vi "CDEx Draw Helicopter 3D Model.vi"(7 "Reset?":bool, 9 "Pitch":dbl, 10 "Travel":dbl, 11 "Elevation":dbl) -> (3 "Scene.New Object":refnum<vi>)   [LabVIEW 2015]
doc: "This VI draws the Flexible Joint using the \"LabVIEW 3D Picture Control Evaluation Software\".\nThe evaluation software can be downloaded from the following URL: http://digital.ni.com/express.nsf/express?openagent&code=exn4gy"
uses:
  <vilib>/picture/3D Picture Control/NI_3D Picture Control.lvlib
panel:
  out "3D Picture Control":refnum<vi>(3d-picture)
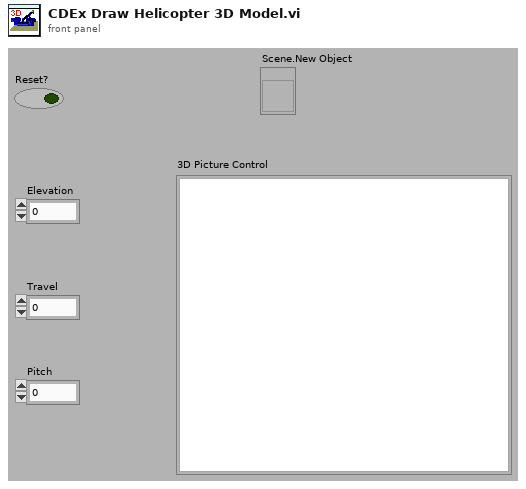
[diagram p1: front panel]
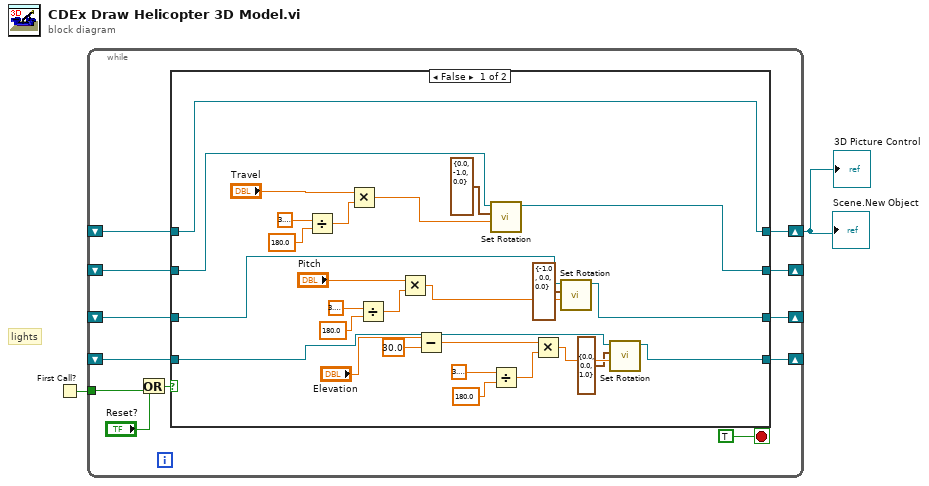
[diagram p0: block diagram]
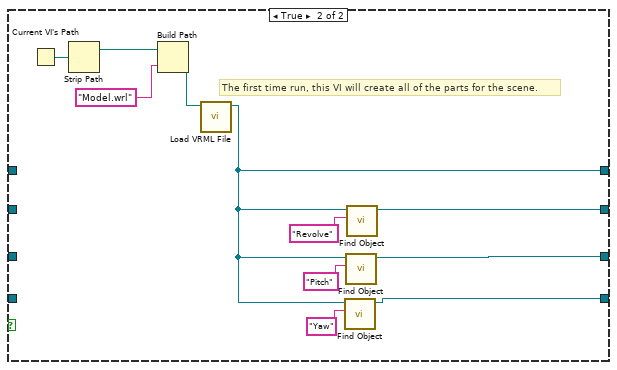
[diagram p2: hidden frame]
diagram:
  # "lights"
  n1 = First Call?() -> (First Call?: T/F=w2:bool)
  n2 = while {
    shift-right: [w6] -> w1
    shift-left: _ -> [w5]
    shift-right: [w13] -> _
    shift-left: _ -> [w12]
    shift-right: [w11] -> _
    shift-left: _ -> [w10]
    tunnel: w2 -> [w7]
    shift-right: [w4] -> _
    shift-left: _ -> [w3]
    stop <- TRUE stop-if-true
    n3 = Or(x="Reset?", y=w7) -> (x .or. y?=w9:bool)
    n4 = case shown="False" w9 {
      tunnel: [w25 w49] -> w13
      tunnel: w12 -> [w27 _]
      tunnel: [w22 w50] -> w11
      tunnel: w10 -> [w23 _]
      tunnel: [w28 w43] -> w6
      tunnel: w5 -> [w28 _]
      tunnel: [w18 w42] -> w4
      tunnel: w3 -> [w17 _]
      frame False {
        n5 = Divide(x=3.141592653589793, y=180.0) -> (x/y=w39:dbl)
        n6 = Multiply(x="Travel", y=w39) -> (x*y=w26:dbl)
        n7 = Divide(x=3.141592653589793, y=180.0) -> (x/y=w36:dbl)
        n8 = Multiply(x="Pitch", y=w36) -> (x*y=w21:dbl)
        n9 = Subtract(x="Elevation", y=30.0) -> (x-y=w30:dbl)
        n10 = call <vilib>:"Set Rotation.vi"("Angle"=w26, "Axis"=cluster{"X":sgl, "Y":sgl, "Z":sgl} {"X"=0.0, "Y"=-1.0, "Z"=0.0}, "Scene Object"=w27) -> ("Rotated Scene Object"=w25:refnum<vi>)  [unwired: 1 in, 7 out]
        n11 = Divide(x=3.141592653589793, y=180.0) -> (x/y=w33:dbl)
        n12 = Multiply(x=w30, y=w33) -> (x*y=w19:dbl)
        n13 = call <vilib>:"Set Rotation.vi"("Angle"=w21, "Axis"=cluster{"X":sgl, "Y":sgl, "Z":sgl} {"X"=-1.0, "Y"=0.0, "Z"=0.0}, "Scene Object"=w23) -> ("Rotated Scene Object"=w22:refnum<vi>)  [unwired: 1 in, 7 out]
        n14 = call <vilib>:"Set Rotation.vi"("Angle"=w19, "Axis"=cluster{"X":sgl, "Y":sgl, "Z":sgl} {"X"=0.0, "Y"=0.0, "Z"=1.0}, "Scene Object"=w17) -> ("Rotated Scene Object"=w18:refnum<vi>)  [unwired: 1 in, 7 out]
      }
      frame True {
        # "The first time run, this VI will create all of the parts for the scene."
        n15 = Current VI's Path() -> (path=w48:path)
        n16 = Strip Path(path=w48) -> (stripped path=w47:path)  [unwired: 1 out]
        n17 = Build Path(base path=w47, name or relative path="Model.wrl") -> (appended path=w45:path)
        n18 = call <vilib>:"Load VRML File.vi"("Path"=w45) -> ("Scene:Read Scene File"=w43:refnum<vi>)  [unwired: 1 in, 9 out]
        n19 = call <vilib>:"Find Object.vi"("Object Name"="Yaw" ("Name"), "Scene Refnum"=w43) -> ("Object Refnum"=w42:refnum<vi>)  [unwired: 1 in, 8 out]
        n20 = call <vilib>:"Find Object.vi"("Object Name"="Pitch" ("Name"), "Scene Refnum"=w43) -> ("Object Refnum"=w50:refnum<vi>)  [unwired: 1 in, 8 out]
        n21 = call <vilib>:"Find Object.vi"("Object Name"="Revolve" ("Name"), "Scene Refnum"=w43) -> ("Object Refnum"=w49:refnum<vi>)  [unwired: 1 in, 8 out]
      }
    }
  }
  "Scene.New Object" <- w1
  "3D Picture Control" <- w1
